vi "MTooltest02.vi"() -> ()   [LabVIEW 2019]
panel:
  out "hex integer string":string
  in  "ChangeStatus":u16(ring) items=["IT8511", "34450A", "WRBuff"]
  in  "Ringfor34450A":u16(ring) items=["SYSTem:VERSion?", "SYSTem:ERRor?", "*IDN?", "MEAS:CURR:DC?", "MEAS:VOLT?", "SYSTem:ERRor?"]
  in  "RingforIT8511":u16(ring) items=["SYSTem:VERSion?", "SYSTem:ERRor?", "*IDN?", "MEAS:CURR:DC?", "MEAS:VOLT?", "MEAS:VOLT:DC?"]
  in  "Boolean 2":bool
  in  "milliseconds to wait":u32
  out "read buffer":string
  in  "write buffer":string
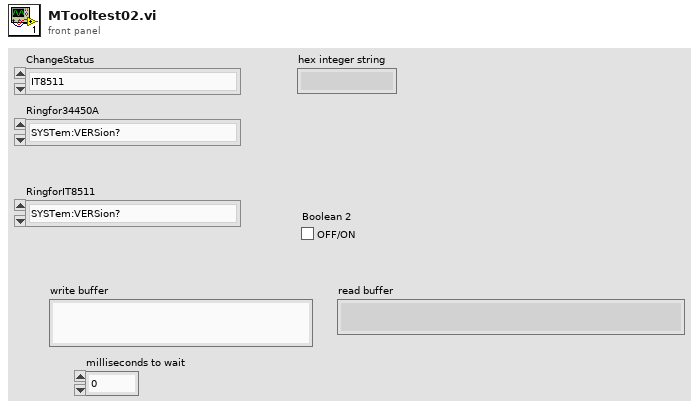
[diagram p1: front panel]
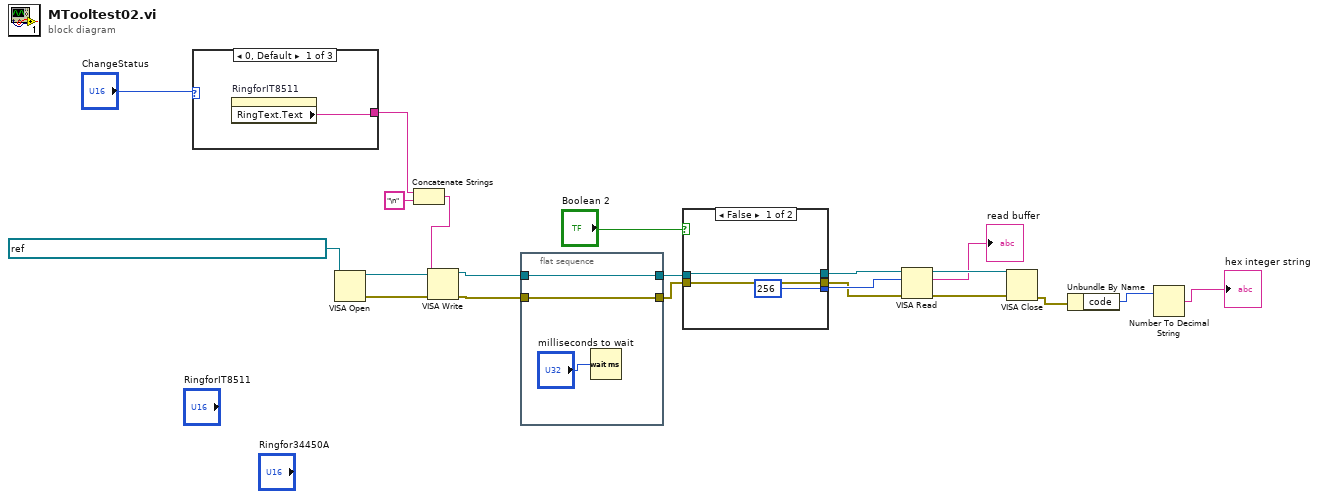
[diagram p0: block diagram]
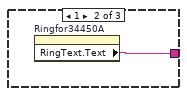
[diagram p2: hidden frame]
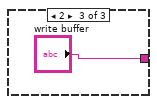
[diagram p3: hidden frame]
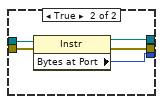
[diagram p4: hidden frame]
diagram:
  n1 = case shown="0, Default" "ChangeStatus" {
    tunnel: [w22 w23 "write buffer"] -> w5
    frame 0, Default {
      n2 = property on="RingforIT8511" class="Ring (strict)"() -> ("RingText.Text"=w22:string)  [unwired: 2 in, 2 out]
    }
    frame 1 {
      n3 = property on="Ringfor34450A" class="Ring (strict)"() -> ("RingText.Text"=w23:string)  [unwired: 2 in, 2 out]
    }
    frame 2 {
    }
  }
  n4 = VISA Open(VISA resource name=refnum<visa-resource-name> "COM3") -> (VISA resource name=w20:refnum<visa-resource-name>, error out=w19:errorcluster)  [unwired: 4 in]
  n5 = Concatenate Strings(w5, "\n" ("string")) -> (w6:string)
  n6 = VISA Write(VISA resource name=w20, write buffer=w6, error in (no error)=w19) -> (VISA resource name out=w12:refnum<visa-resource-name>, error out=w16:errorcluster)  [unwired: 1 out]
  n7 = flat-sequence {
    tunnel: w16 -> [w26]
    tunnel: [w26] -> w11
    tunnel: [w25] -> w13
    tunnel: w12 -> [w25]
    frame #0 {
      n8 = Wait (ms)(milliseconds to wait="milliseconds to wait") -> ()  [unwired: 1 out]
    }
  }
  n9 = case shown="False" "Boolean 2" {
    tunnel: [u32 256 ("Bytes at Port") w35] -> w14
    tunnel: w13 -> [w30 w34]
    tunnel: w11 -> [w29 w33]
    tunnel: [w29 w32] -> w10
    tunnel: [w30 w31] -> w9
    frame False {
    }
    frame True {
      n10 = property class="Instr"(reference=w34, error in=w33) -> (reference out=w31:refnum<visa-resource-name>, error out=w32:errorcluster, "Bytes at Port"=w35:u32)
    }
  }
  n11 = VISA Read(VISA resource name=w9, byte count=w14, error in (no error)=w10) -> (VISA resource name out=w18:refnum<visa-resource-name>, read buffer=→"read buffer":string, error out=w17:errorcluster)  [unwired: 1 out]
  n12 = VISA Close(VISA resource name=w18, error in (no error)=w17) -> (error out=w3:errorcluster)
  n13 = Unbundle By Name(w3) -> ("code"=w2:i32)
  n14 = Number To Decimal String(number=w2) -> (decimal integer string=→"hex integer string":string)  [unwired: 1 in]
